vi "sequence file utility.vi"() -> ()   [LabVIEW 2021]
panel:
  in  "include sequences in the same folder and subfolder":bool
  in  "path of \"a\" sequence file":path=path "C:/Users/shared/Sequences/Thermal conductivity/SCM2_fast_Hsweepdn.txt"
  in  "overwrite?":bool=TRUE
  in  "find and replace":T1(array[cluster])=[{"replace this"="Set Parameter", "with this"="Set Parameter localhost,"}, {"replace this"="Wait for VI value", "with this"="Wait for VI value localhost,"}, {"replace this"="Run VI:", "with this"="Run VI: localhost,"}, {"replace this"="Abort VI:", "with this"="Abort VI: localhost,"}]
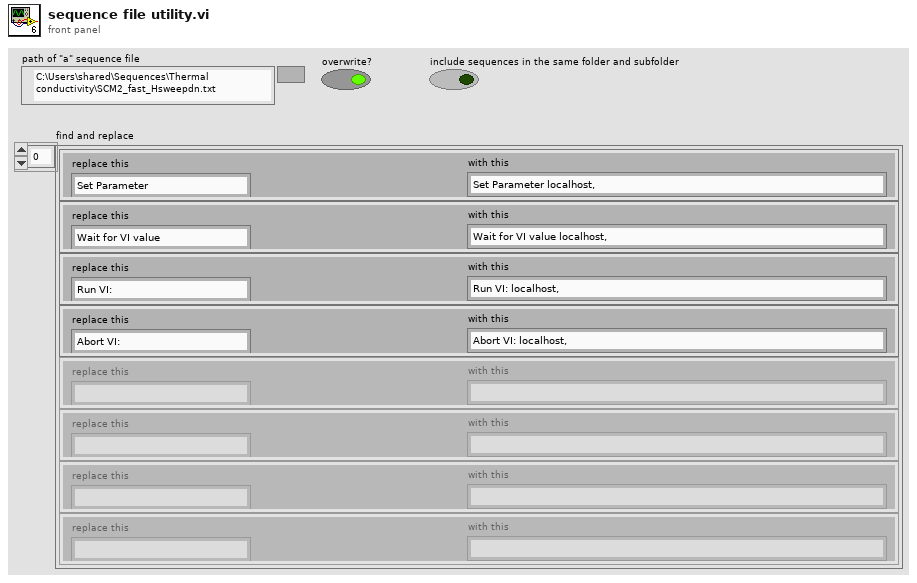
[diagram p1: front panel]
types:
  T1 = cluster{"replace this":string, "with this":string}[]
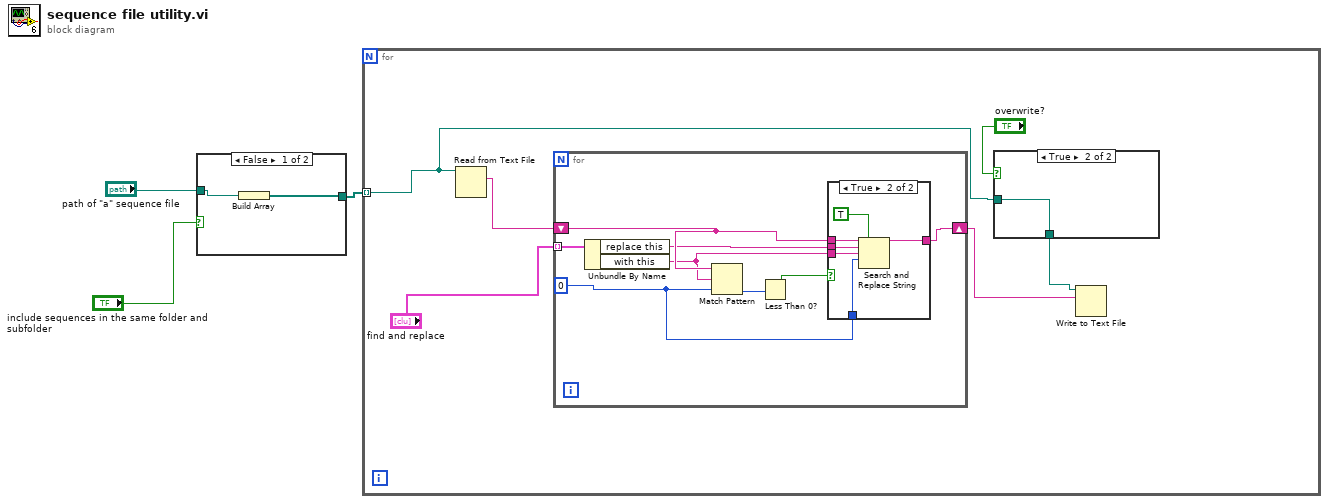
[diagram p0: block diagram]
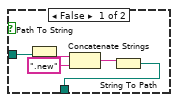
[diagram p2: hidden frame]
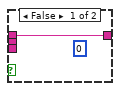
[diagram p3: hidden frame]
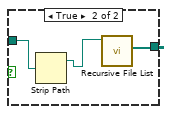
[diagram p4: hidden frame]
diagram:
  n1 = case shown="False" "include sequences in the same folder and subfolder" {
    tunnel: "path of \"a\" sequence file" -> [w5 w7]
    tunnel: [w4 w8] -> w1
    frame False {
      n2 = Build Array(w5) -> (w4:path[])
    }
    frame True {
      n3 = Strip Path(path=w7) -> (stripped path=w6:path)  [unwired: 1 out]
      n4 = call <vilib>:"Recursive File List.vi"("Folder Path"=w6) -> ("All Files in Dir"=w8:path[])  [unwired: 6 in, 4 out]
    }
  }
  n5 = for {
    tunnel: w1 -> [w9] mode=indexing
    n6 = Read from Text File(file (use dialog)=w9) -> (text=w14:string)  [unwired: 3 in, 3 out]
    n7 = for {
      tunnel: "find and replace" -> [w28] mode=indexing
      shift-right: [w26] -> w12
      shift-left: w14 -> [w27]
      w24 = 0 ("offset past replacement")
      n8 = Unbundle By Name(w28) -> ("replace this"=w22:string, "with this"=w21:string)
      n9 = Match Pattern(string=w27, regular expression=w21, offset (0)=w24) -> (offset past match=w23:i32)  [unwired: 3 out]
      n10 = Less Than 0?(x=w23) -> (x < 0?=w25:bool)
      n11 = case shown="True" w25 {
        tunnel: w27 -> [w29 w35]
        tunnel: w22 -> [_ w34]
        tunnel: w21 -> [_ w33]
        tunnel: [w29 w32] -> w26
        tunnel: w24 -> [_ w31]
        frame False {
          (unwired) 0 ("number of replacements")
        }
        frame True {
          n12 = Search and Replace String(replace all?=TRUE ("replace all? (F)"), input string=w35, search string=w34, replace string=w33, offset=w31) -> (result string=w32:string)  [unwired: 3 in, 3 out]
        }
      }
    }
    n13 = case shown="True" "overwrite?" {
      tunnel: [w15 w20] -> w10
      tunnel: w9 -> [w19 w20]
      frame False {
        n14 = Path To String(path=w19) -> (string=w18:string)
        n15 = Concatenate Strings(w18, ".new" ("string")) -> (w16:string)
        n16 = String To Path(string=w16) -> (path=w15:path)
      }
      frame True {
      }
    }
    n17 = Write to Text File(file (use dialog)=w10, text=w12) -> ()  [unwired: 2 in, 3 out]
  }
